vi "WM Regular Wave Settings for IO.vi"(1 "Settings":T1={"Output Device"=1, "Output Channel"="0", "Sampling Rate (Hz)"=200.0, "Input Device"=1, "Input Channel"="0", "Input Offset (V)"=0.0, "Input Calibration (m/V)"=1.0, "Stroke Calibration (V/m)"=7.8564, "Paddle Height (m)"=3.3147, "Water Depth (m)"=2.44, "Min Period"=0.5, "Max Period"=5.0, "Max 1/2 Piston Stroke"=0.16, "Max H/L"=0.1, "Max H/d"=0.65} {"Input Calibration (m/V)" format="%.4f"; "Input Offset (V)" format="%.4f"; "Max H/d" format="%.2f"; "Max H/L" format="%.2f"; "Max 1/2 Piston Stroke" format="%.2f"; "Max Period" format="%.2f"; "Min Period" format="%.2f"; "Water Depth (m)" format="%.2f"; "Paddle Height (m)" format="%.4f"; "Stroke Calibration (V/m)" format="%.4f"; "Sampling Rate (Hz)" format="%.2f"}) -> (0 "Settings Output":T1={"Output Device"=1, "Output Channel"="0,1", "Sampling Rate (Hz)"=50.0, "Input Device"=1, "Input Channel"="0", "Input Offset (V)"=0.0, "Input Calibration (m/V)"=1.0, "Stroke Calibration (V/m)"=7.8564, "Paddle Height (m)"=3.3147, "Water Depth (m)"=2.44, "Min Period"=0.5, "Max Period"=5.0, "Max 1/2 Piston Stroke"=0.16, "Max H/L"=0.1, "Max H/d"=0.65} {"Input Calibration (m/V)" format="%.2f"; "Input Offset (V)" format="%.2f"; "Max H/d" format="%.2f"; "Max H/L" format="%.2f"; "Max 1/2 Piston Stroke" format="%.2f"; "Max Period" format="%.2f"; "Min Period" format="%.2f"; "Water Depth (m)" format="%.2f"; "Paddle Height (m)" format="%.4f"; "Stroke Calibration (V/m)" format="%.4f"; "Sampling Rate (Hz)" format="%.2f"})   [LabVIEW 2012]
panel:
  in  "OK":bool=TRUE
  # "Input / Output"
  # "Limits"
  # "Input / Output"
  # "Limits"
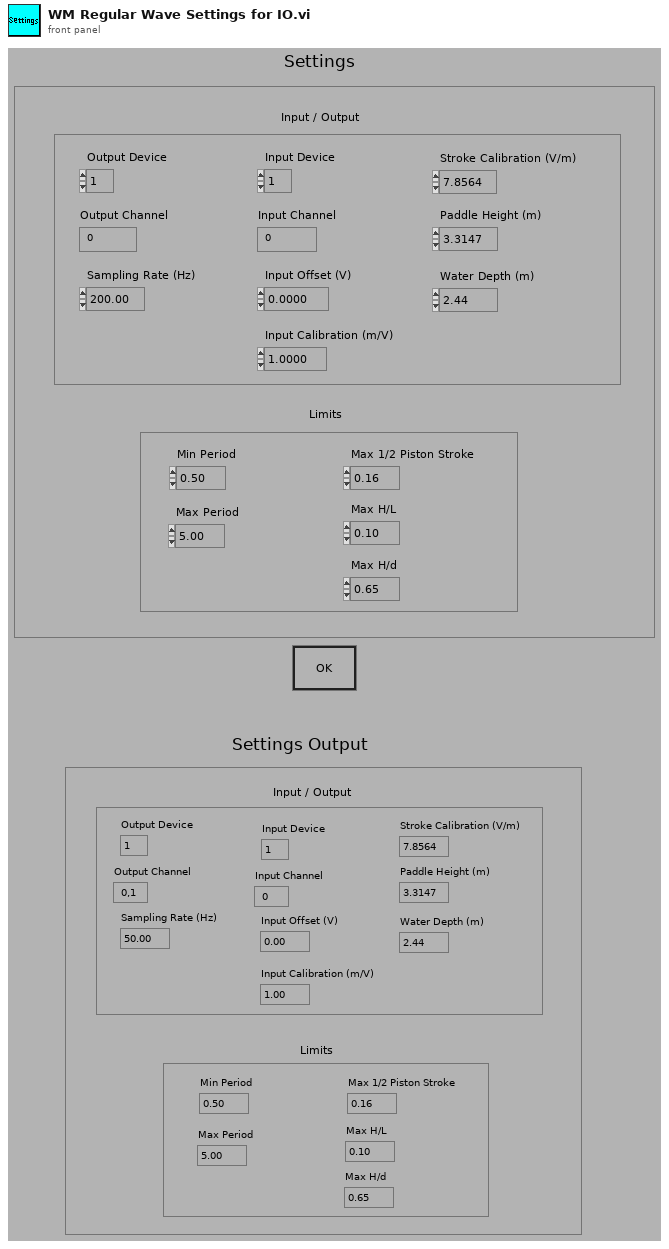
[diagram p1: front panel]
types:
  T1 = cluster{"Output Device":i16, "Output Channel":string, "Sampling Rate (Hz)":dbl, "Input Device":i16, "Input Channel":string, "Input Offset (V)":dbl, "Input Calibration (m/V)":dbl, "Stroke Calibration (V/m)":dbl, "Paddle Height (m)":dbl, "Water Depth (m)":dbl, "Min Period":dbl, "Max Period":dbl, "Max 1/2 Piston Stroke":dbl, "Max H/L":dbl, "Max H/d":dbl}
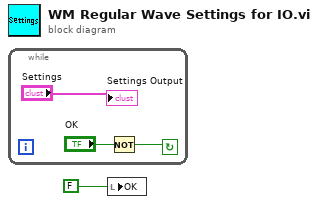
[diagram p0: block diagram]
diagram:
  n1 = while {
    stop <- w3 continue-if-true
    n2 = Not(x="OK") -> (.not. x?=w3:bool)
    "Settings Output" <- "Settings"
  }
  n3 = local write "OK"(FALSE ("OK")) -> ()
